vi "ExposeConvertObjectMapDataValueToVartiant.vi"(9 "Allow Variant Values (f)":bool, 10 "NamepathData":T1, 11 "Data Value":variant) -> (3 "Value Ref":refnum<data-value>)   [LabVIEW 2017]
uses:
  ExposeMapperDataTypeEnum.ctl
  ExposeObjectMapNamepathData.ctl
  ExposeObjectMapContainerTypeEnum.ctl
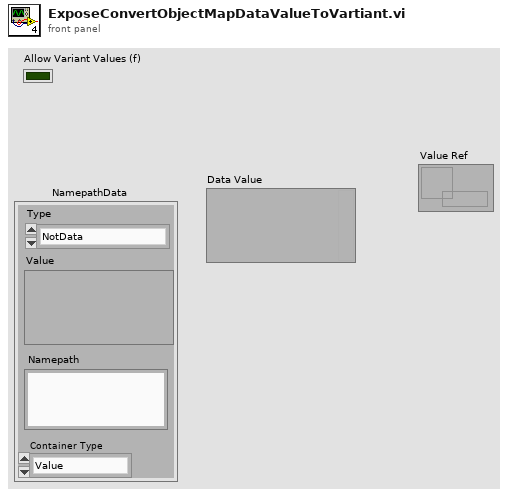
[diagram p1: front panel]
types:
  T1 = typedef "ExposeObjectMapNamepathData.ctl" = cluster{"Type":T2, "Value":variant, "Namepath":string, "Container Type":T3}
  T2 = typedef "ExposeMapperDataTypeEnum.ctl" = enum16{"NotData", "int8", "byte", "int16", "uint16", "int32", "uint32", "int64", "uint64", "Single", "Double", "String", "Boolean", "Container"}
  T3 = typedef "ExposeObjectMapContainerTypeEnum.ctl" = enum16{"Value", "Array", "Waveform", "NetContainer"}
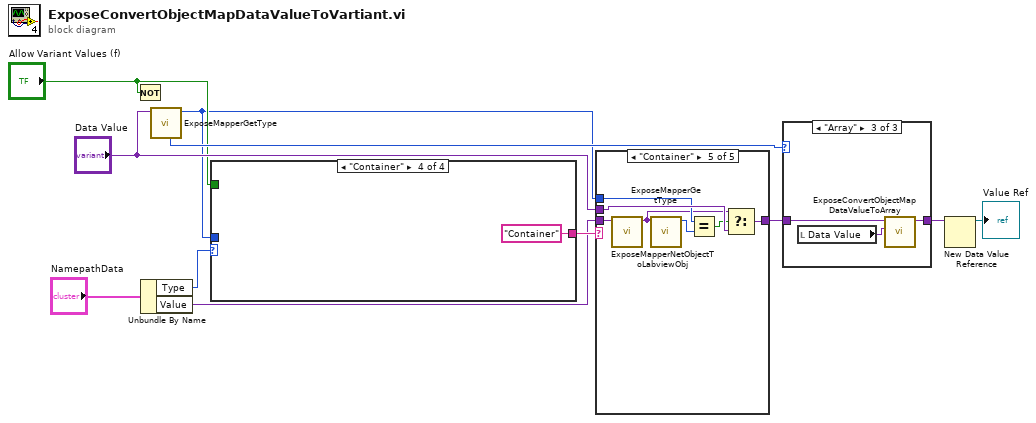
[diagram p0: block diagram]
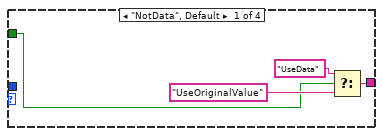
[diagram p2: hidden frame]
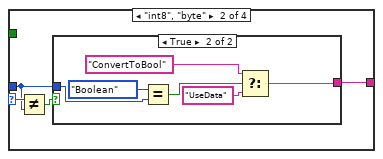
[diagram p3: hidden frame]
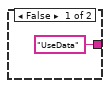
[diagram p4: hidden frame]
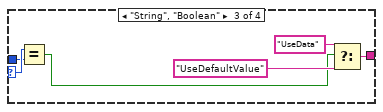
[diagram p5: hidden frame]
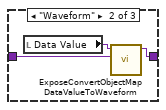
[diagram p7: hidden frame]
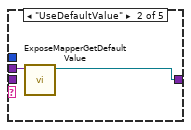
[diagram p9: hidden frame]
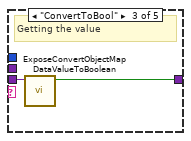
[diagram p10: hidden frame]
diagram:
  n1 = Not(x="Allow Variant Values (f)") -> ()  [unwired: 1 out]
  n2 = Unbundle By Name("NamepathData") -> ("Type"=w4:T2, "Value"=w5:variant)
  n3 = call "ExposeMapperGetType.vi"("Data Val Ref in"="Data Value") -> ("DataType"=w3:T2, "Container Type (Labview Value type)"=w8:T3)  [unwired: 5 in, 4 out]
  n4 = case shown="\"Container\"" w4 {
    selector: w4 -> [_ w19 w32 _]
    tunnel: [w12 w17 w27 "Container"] -> w6
    tunnel: w3 -> [_ w16 w31 _]
    tunnel: "Allow Variant Values (f)" -> [w14 _ _ _]
    frame "NotData", Default {
      n5 = Select(t="UseData", s=w14, f="UseOriginalValue") -> (s? t:f=w12:string)
    }
    frame "int8", "byte" {
      n6 = Not Equal?(x=w19, y=w16) -> (x != y?=w18:bool)
      n7 = case shown="True" w18 {
        tunnel: ["UseData" w21] -> w17
        tunnel: w16 -> [_ w26]
        frame False {
        }
        frame True {
          n8 = Equal?(x=ExposeMapperDataTypeEnum."Boolean", y=w26) -> (x = y?=w24:bool)
          n9 = Select(t="ConvertToBool", s=w24, f="UseData") -> (s? t:f=w21:string)
        }
      }
    }
    frame "String", "Boolean" {
      n10 = Equal?(x=w32, y=w31) -> (x = y?=w29:bool)
      n11 = Select(t="UseData", s=w29, f="UseDefaultValue") -> (s? t:f=w27:string)
    }
    frame "Container" {
    }
  }
  n12 = case shown="\"Container\"" w6 {
    tunnel: [w34 w36 w38 w39 w40] -> w11
    tunnel: "Data Value" -> [_ w35 _ w39 w45]
    tunnel: w5 -> [w34 _ w37 _ w46]
    tunnel: w3 -> [_ _ _ _ w44]
    frame Default {
    }
    frame "UseDefaultValue" {
      n13 = call "ExposeMapperGetDefaultValue.vi"("Data Val Ref in"=w35) -> ("Data Val Ref Out"=w36:refnum<data-value>)  [unwired: 10 in]
    }
    frame "ConvertToBool" {
      # "Getting the value"
      n14 = call "ExposeConvertObjectMapDataValueToBoolean.vi"("Data Value"=w37) -> ("Boolean"=w38:bool)  [unwired: 10 in]
    }
    frame "UseOriginalValue" {
    }
    frame "Container" {
      n15 = call "ExposeMapperNetObjectToLabviewObj.vi"("Value"=w46) -> ("variant"=w42:variant)  [unwired: 10 in]
      n16 = call "ExposeMapperGetType.vi"("Data Val Ref in"=w42) -> ("DataType"=w43:T2)  [unwired: 5 in, 5 out]
      n17 = Equal?(x=w44, y=w43) -> (x = y?=w41:bool)
      n18 = Select(t=w42, s=w41, f=w45) -> (s? t:f=w40:variant)
    }
  }
  n19 = case shown="\"Array\"" w8 {
    tunnel: w11 -> [w47 w50 w52]
    tunnel: [w47 w48 w53] -> w2
    frame Default {
    }
    frame "Waveform" {
      n20 = local read "Data Value"() -> (w49:variant)
      n21 = call "ExposeConvertObjectMapDataValueToWaveform.vi"("Numbers Vector"=w50, "Waveform"=w49) -> ("Data Value out"=w48:variant)  [unwired: 9 in]
    }
    frame "Array" {
      n22 = local read "Data Value"() -> (w51:variant)
      n23 = call "ExposeConvertObjectMapDataValueToArray.vi"("Original Value"=w51, "Data"=w52) -> ("Array"=w53:variant)  [unwired: 9 in]
    }
  }
  n24 = New Data Value Reference(data value=w2) -> (data value reference=→"Value Ref":refnum<data-value>)  [unwired: 1 in, 1 out]
